vi "StreamErrorFilter.vi"(8 "error in (no error)":errorcluster) -> (0 "error out":errorcluster)   [LabVIEW 2017]
uses:
  <vilib>/ErrorRing/Error Ring.xnode
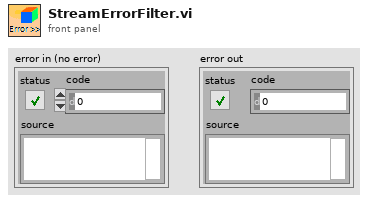
[diagram p1: front panel]
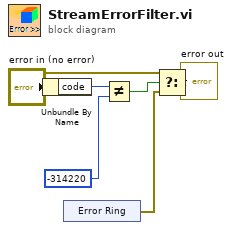
[diagram p0: block diagram]
diagram:
  n1 = Unbundle By Name("error in (no error)") -> ("code"=w2:i32)
  n2 = xnode "Error Ring"() -> ("error out"=w5:errorcluster)
  n3 = Not Equal?(x=w2, y=-314220) -> (x != y?=w4:bool)
  n4 = Select(t="error in (no error)", s=w4, f=w5) -> (s? t:f=→"error out":errorcluster)
